vi "Read Configuration File.vi"(8 "error in (no error)":errorcluster, 11 "Example Instrument in":refnum<class "Instrument.FrameworkTemplate.lvclass">) -> (0 "error out":errorcluster, 3 "Example Instrument out":refnum<class "Instrument.FrameworkTemplate.lvclass">)   [LabVIEW 2019, in "Instrument.FrameworkTemplate.lvclass"]
uses:
  Instrument.FrameworkTemplate.lvclass
  C:/Program Files (x86)/National Instruments/LabVIEW 2019/user.lib/LevyLab/Instrument Framework/SMOs/Instrument/Instrument.lvclass
  <userlib>/LevyLab/Instrument Framework/SMOs/Instrument/Instrument.lvclass/Instrument.ctl
  <userlib>/LevyLab/Instrument Framework/SMOs/Configuration/Configuration.lvclass/Configuration.ctl
  Instrument.FrameworkTemplate.lvclass/Instrument.FrameworkTemplate.ctl
  <userlib>/LevyLab/Instrument Framework/SMOs/Configuration/Write Section.vi
  <userlib>/LevyLab/Instrument Framework/SMOs/Instrument/Instrument.lvclass
  C:/Program Files (x86)/National Instruments/LabVIEW 2019/vi.lib/JKI/JKI SMO/SMO/SMO.lvclass
  <vilib>/JKI/JKI SMO/SMO/Protected/ThisLevelClassName.vi
  <userlib>/LevyLab/Instrument Framework/Instrument Types/VSource/Instrument.VSource.lvclass
  <userlib>/LevyLab/Instrument Framework/SMOs/Configuration/Configuration.lvclass
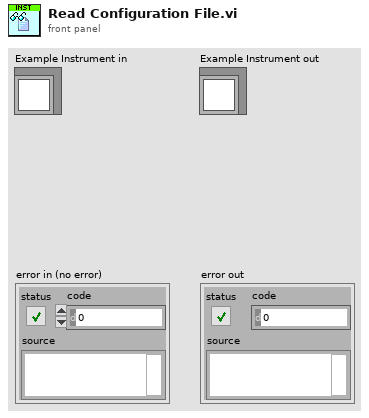
[diagram p1: front panel]
types:
  T1 = typedef "Instrument.FrameworkTemplate.lvclass/Instrument.FrameworkTemplate.Configuration--Cluster.ctl" = cluster{"Example Setting 1":dbl, "Example Setting 2":dbl, "Example Setting 3":string}
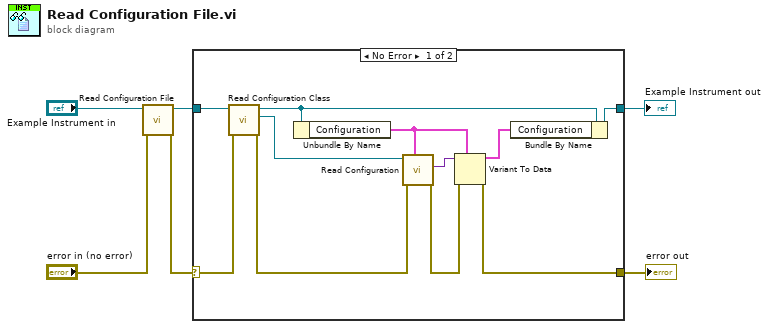
[diagram p0: block diagram]
diagram:
  n1 = call-parent "Read Configuration File.vi"("error in (no error)"="error in (no error)", "Instrument in"="Example Instrument in") -> ("error out"=w2:errorcluster, "Instrument out"=w1:refnum<class "Instrument.FrameworkTemplate.lvclass">)  [unwired: 8 in]
  n2 = case shown="No Error" w2 {
    selector: w2 -> [w13 w19]
    tunnel: w1 -> [w15 w18]
    tunnel: [w11 w18] -> w6
    tunnel: [w14 w19] -> w5
    frame No Error {
      n3 = call <userlib>:"Read Configuration Class.vi"("error in (no error)"=w13, "Instrument in"=w15) -> ("error out"=w16:errorcluster, "Configuration"=w7:refnum<class "Configuration.lvclass">, "Instrument out"=w10:refnum<class "Instrument.FrameworkTemplate.lvclass">)  [unwired: 7 in]
      n4 = Unbundle By Name(w10) -> ("Configuration"=w12:T1)
      n5 = call <userlib>:"Read Configuration.vi"("INI Fomatted Cluster Type"=w12, "error in (no error)"=w16, "Configuration in"=w7) -> ("error out"=w17:errorcluster, "Configuration"=w9:variant)  [unwired: 6 in, 1 out]
      n6 = Variant To Data(error in=w17, type=w12, Variant=w9) -> (data=w8:T1, error out=w14:errorcluster)
      n7 = Bundle By Name(cluster=w10, "Configuration"=w8) -> (w11:refnum<class "Instrument.FrameworkTemplate.lvclass">)
    }
    frame Error {
    }
  }
  "Example Instrument out" <- w6
  "error out" <- w5
